vi "2d 10Be.vi"(6 "data in":T6={"Total counts"=0, "cps"=0.0, "live time"=0.0, "pulser"=0.0, "rare counts"=0.0, "other counts"=0.0, "total run time(sec)"=0.0, "adjusted run time(sec)"=0.0, "17O average"=1.0, "17O current"=1.0}, 8 "error in":errorcluster, 9 "1d state control":T7) -> (4 "data out":T6={"Total counts"=0, "cps"=0.0, "live time"=0.0, "pulser"=0.0, "rare counts"=0.0, "other counts"=0.0, "total run time(sec)"=0.0, "adjusted run time(sec)"=0.0, "17O average"=1.0, "17O current"=1.0})   [LabVIEW 2016]
doc: "uses gated region to gather and parse 1d data"
uses:
  controls/1d/1d state event control.ctl
  spectrum/controls/count control.ctl
  controls/display spectrum.ctl
  pixie2d/controls/1d gate selection.ctl
  <vilib>/DAQmx/read.llb/DAQmx Read (Analog 1D DBL 1Chan NSamp).vi
  <vilib>/Analysis/baseanly.llb/Mean (DBL).vi
  <vilib>/DAQmx/miscellaneous.llb/DAQmx Fill In Error Info.vi
  Drivers/Pixie4DLL.dll
  <vilib>/Analysis/NI_AALBase.lvlib
panel:
  out "number of events":dbl
  out "Run time [s]":dbl
  out "run data output":T1
  in  "wait time(milliseconds)":i32=500
  in  "17O scale (nA/V)":dbl=5.0
  out "17O":dbl
  out "error out":errorcluster
  out "17 Average":dbl format="%0.6f"
  out "17O information":dbl[](array[numeric])
  out "sum  17O":dbl format="%0.2f"
  out "splice time":u32 format="%.2e"
  out "17O":dbl(graph)
  in  "1d gate":T3={"channel number"="", "min"=0.0, "max"=32000.0}
  in  "stop":bool
  in  "number of gated regions":i32=3
  in  "spectrum 2":T4 items=["pulser", "gated region 1", "gated region 2", "gated region 3"]
  in  "spectrum":T4 items=["pulser", "gated region 1", "gated region 2", "gated region 3"]
  out "gate 2":dbl[][](graph)
  out "gate 1":dbl[][](graph)
  out "display array out":T5(array[cluster])
  out "Pixie4DLL calls error":errorcluster
  out "run time":sgl
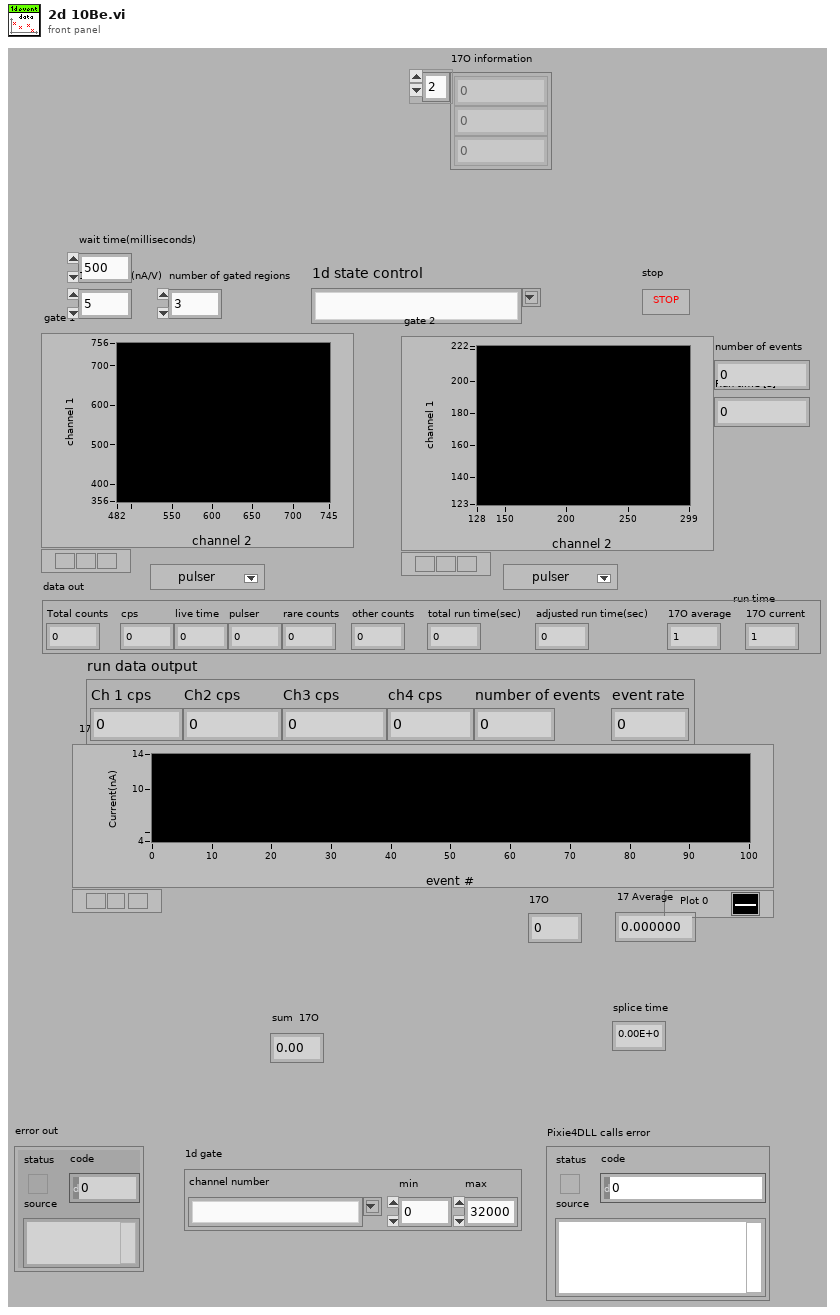
[diagram p1: front panel]
types:
  T1 = cluster{"Ch 1 cps":dbl, "Ch2 cps":dbl, "Ch3 cps":dbl, "ch4 cps":dbl, "number of events":dbl, "event rate":dbl}
  T2 = typedef "1d gate selection.ctl" = string
  T3 = cluster{"channel number":T2, "min":dbl, "max":dbl}
  T4 = typedef "display spectrum.ctl" = u16
  T5 = cluster{"X name":string, "Y name ":string, "counts":dbl, "gate 1":dbl[][], "count rate":dbl, "X Peak":dbl, "Y Peak":dbl, "cathode position":dbl}[]
  T6 = typedef "count control.ctl" = cluster{"Total counts":u32, "cps":dbl, "live time":dbl, "pulser":dbl, "rare counts":dbl, "other counts":dbl, "total run time(sec)":dbl, "adjusted run time(sec)":dbl, "17O average":dbl, "17O current":dbl}
  T7 = typedef "1d state event control.ctl" = string
  T8 = cluster{"X name":string, "Y name ":string, "counts":dbl, "gate 1":dbl[][], "count rate":dbl, "X Peak":dbl, "Y Peak":dbl, "cathode position":dbl}
  T9 = cluster{"input count rate 0":dbl, "input count rate 1":dbl, "input count rate 2":dbl, "input count rate 3":dbl, "number of events":dbl, "event rate":dbl}
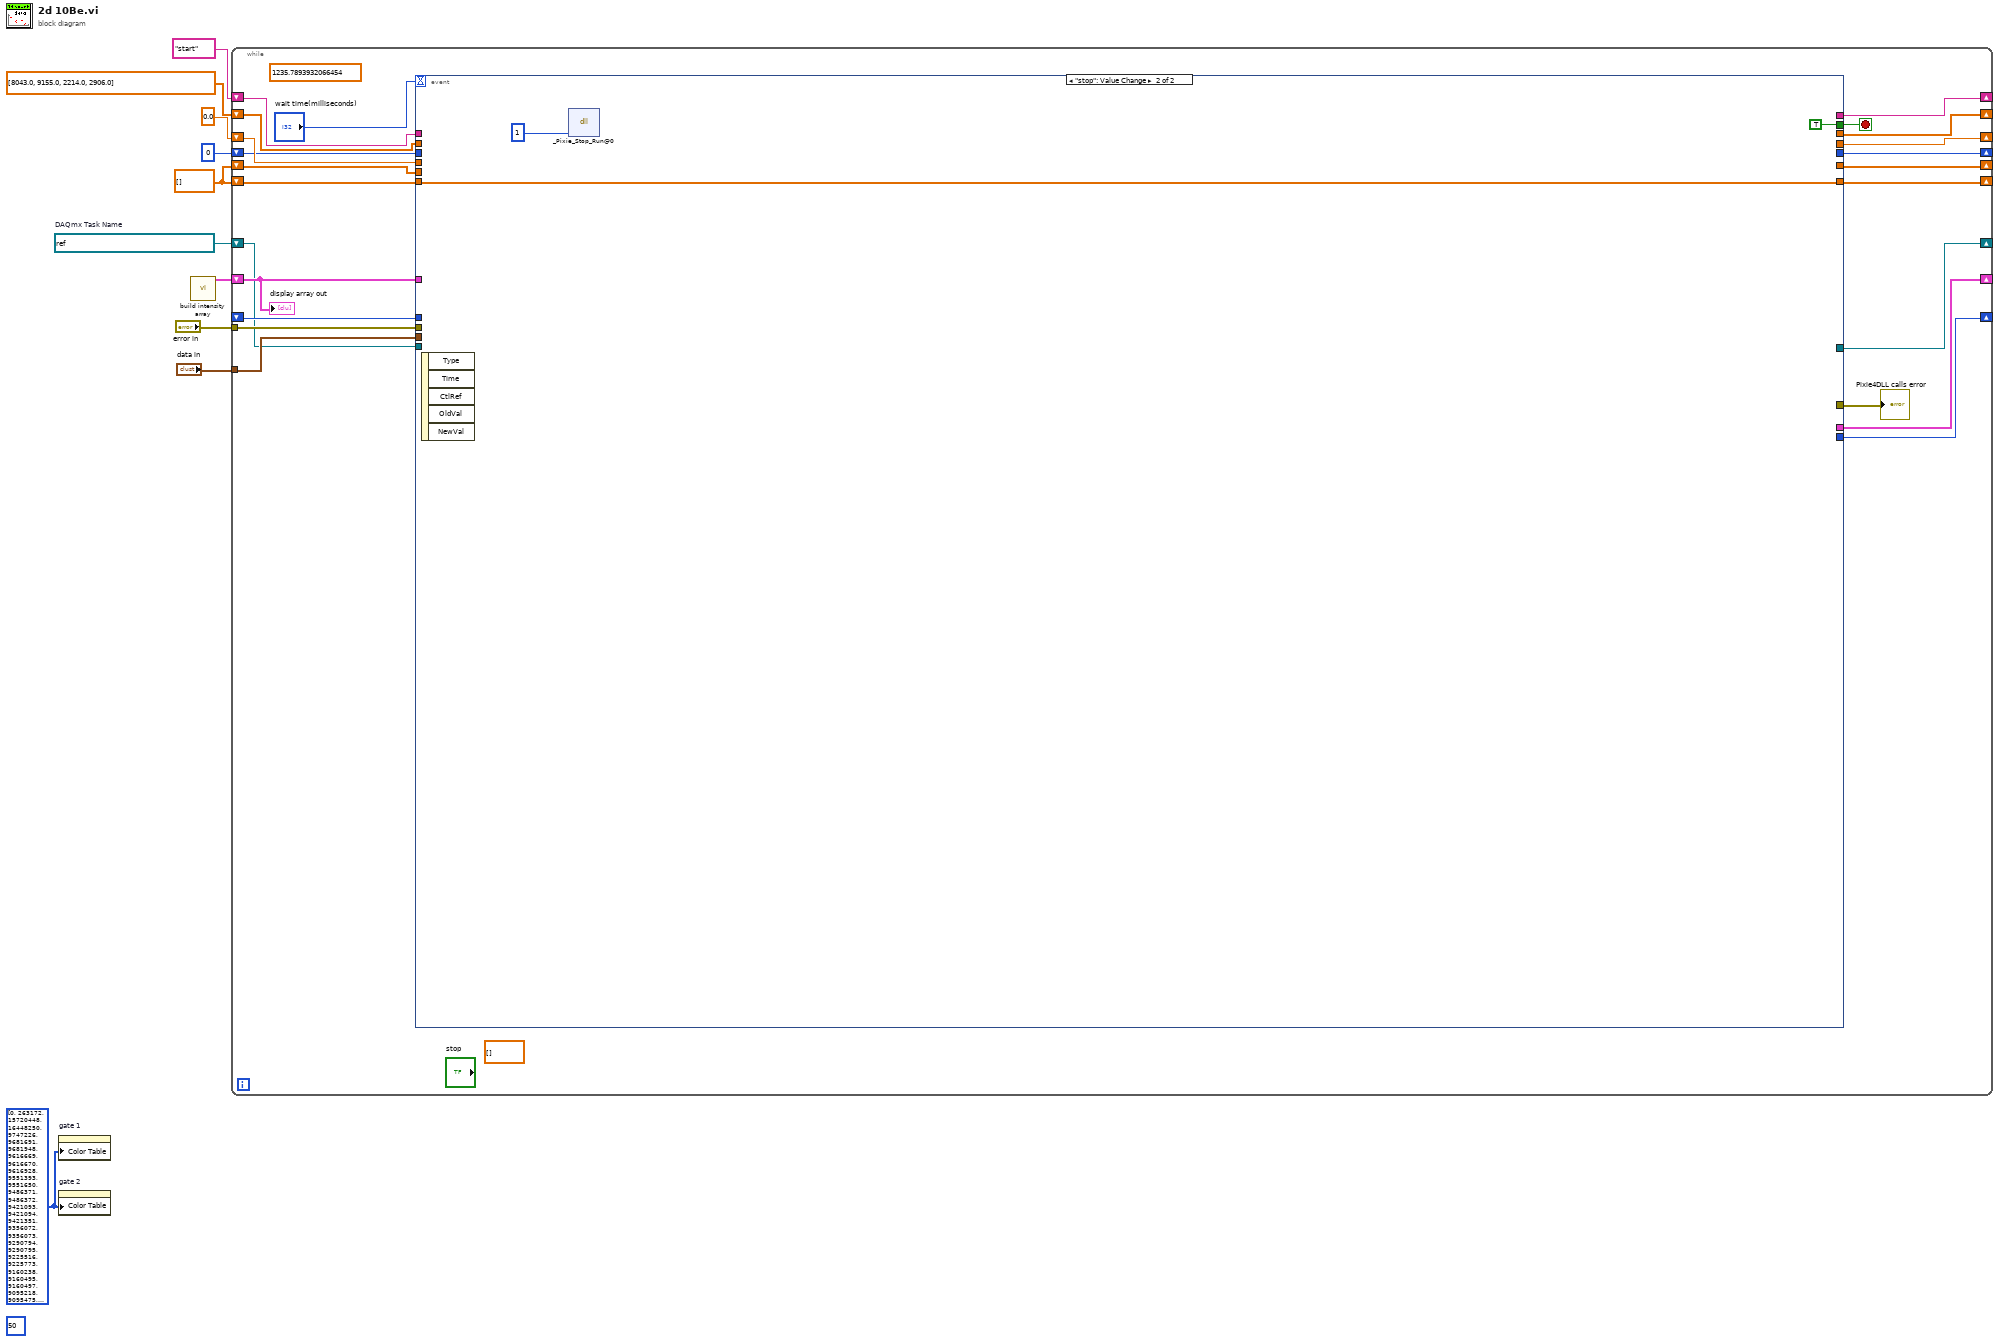
[diagram p0: block diagram]
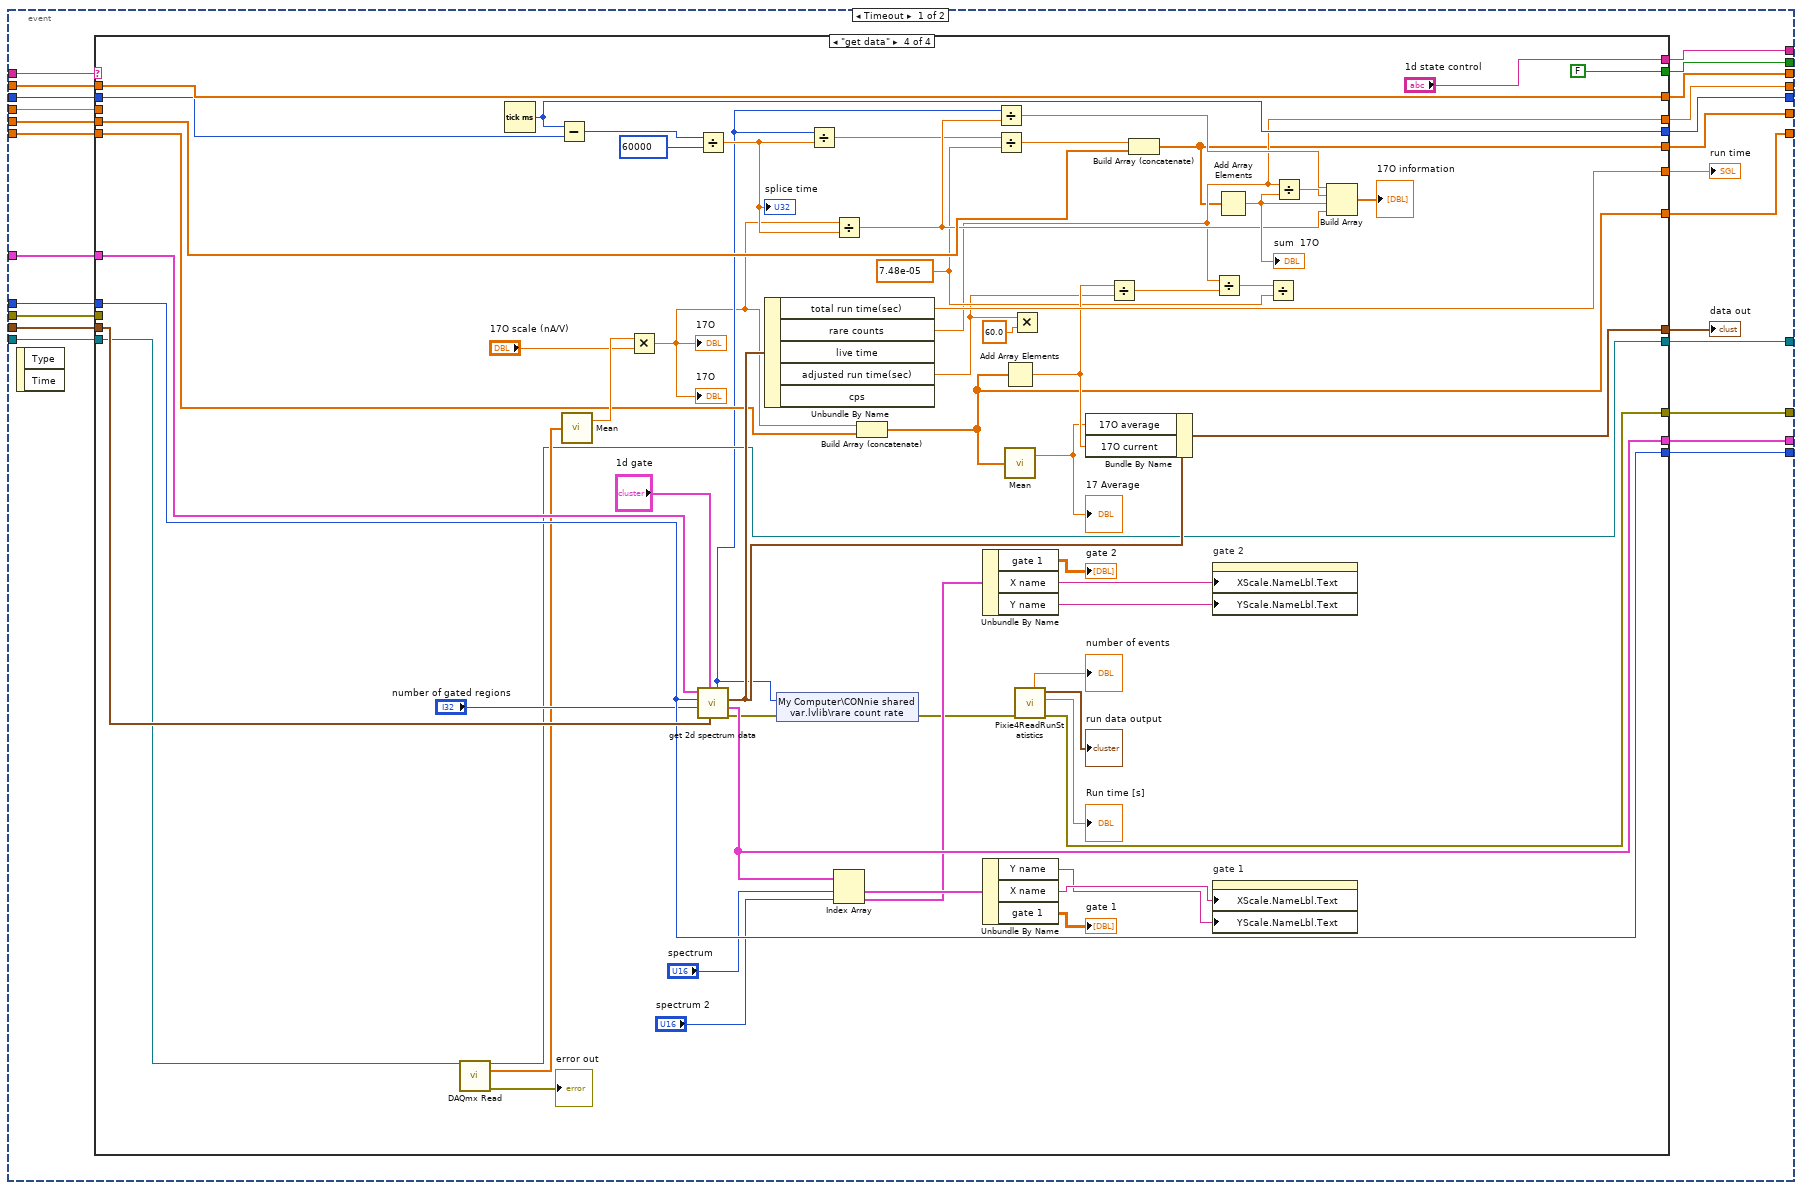
[diagram p2: hidden frame]
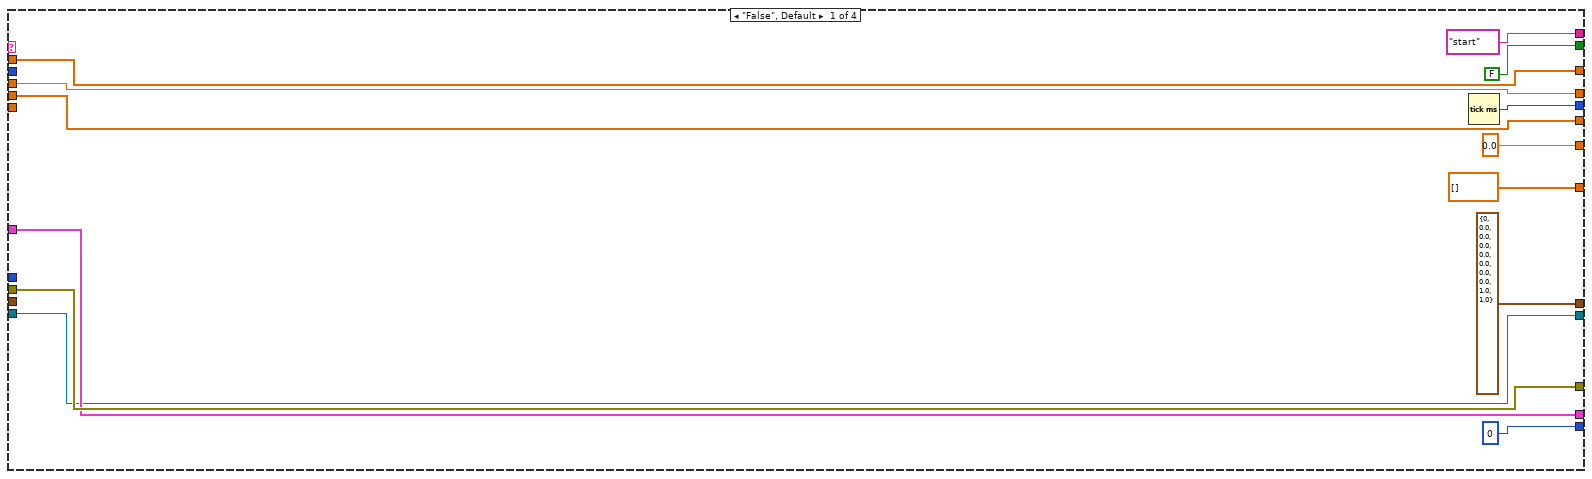
[diagram p3: hidden frame]
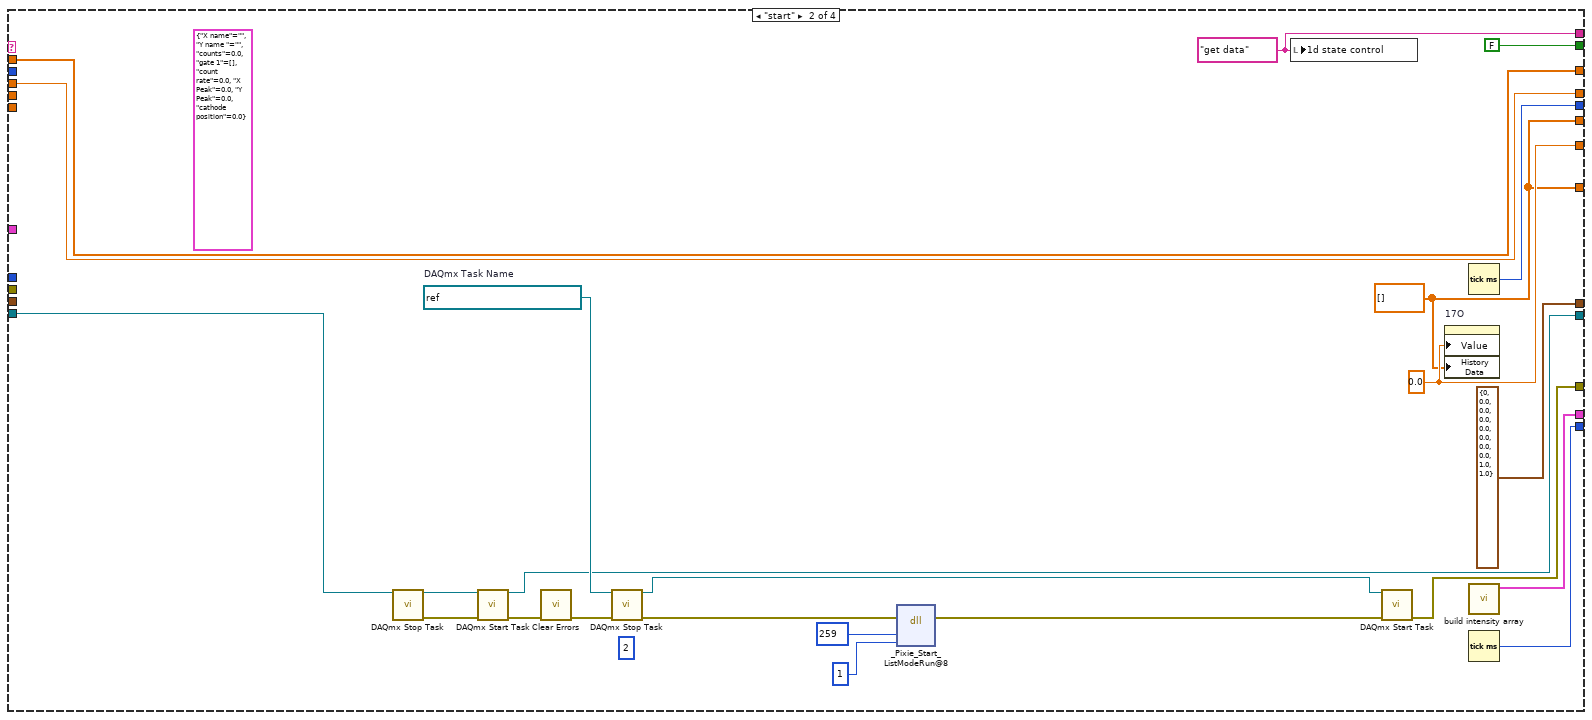
[diagram p4: hidden frame]
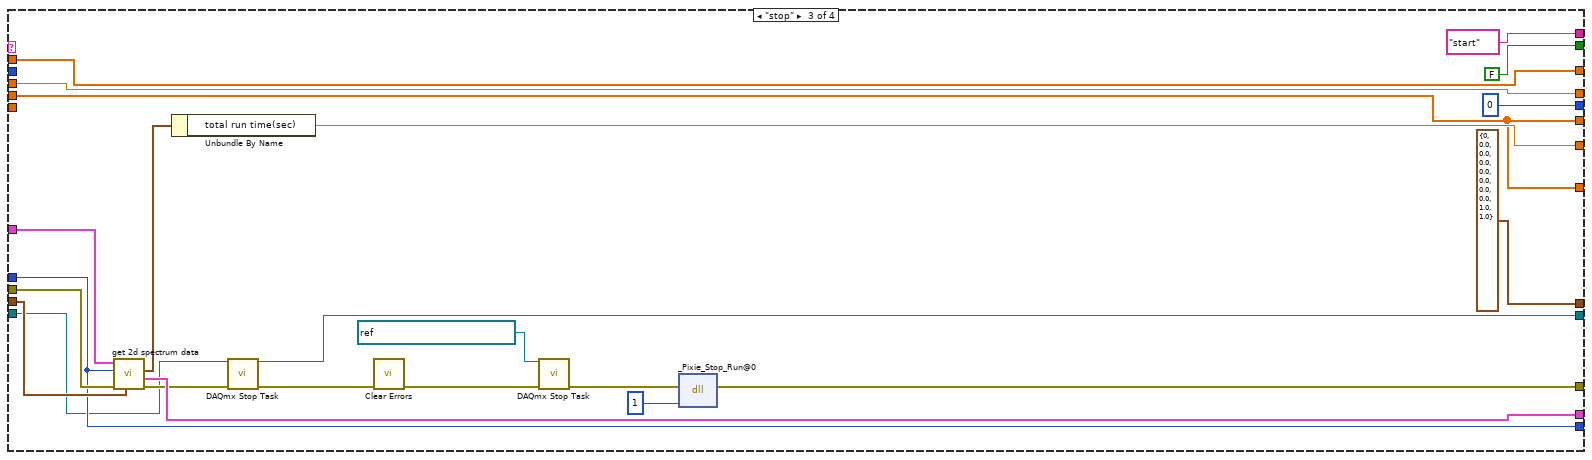
[diagram p5: hidden frame]
diagram:
  w1 = dbl[] []
  w3 = refnum<k21> "measure constant voltage"  # DAQmx Task Name
  w5 = u32[] [0, 263172, 15720448, 16448250, 9747226, 9681691, 9681948, 9616669, 9616670, 9616928, 9551393, 9551650, 9486371, 9486372, 9421093, 9421094, 9421351, 9356072, 9356073, 9290794, 9290795, 9225516, 9225773, 9160238, 9160495, 9160497, 9095218, 9095475, 9029940, 9030197, 8964918, 8964919, 8965176, 8899641, 8899898, 8834619, 8834620, 8769341, 8769342, 8769599, 8704321, 8704322, 8639043, 8639044, 8573765, 8574022, 8574023, 8508744, 8508745, 8443466, 8443723, 8378188, 8378445, 8312910, 8313167, 8312912, 8247122, 8246867, 8181076, 8181077, 8115286, 8115031, 8114776, 8048985, 8048730, 7982939, 7982684, 7916893, 7916894, 7916639, 7850848, 7850594, 7784803, 7784548, 7718757, 7718502, 7718503, 7652712, 7652457, 7586666, 7586411, 7520620, 7520365, 7454574, 7454319, 7454320, 7388529, 7388275, 7322484, 7322229, 7256438, 7256183, 7255928, 7190137, 7190138, 7124347, 7124092, 7058301, 7058046, 7057791, 6992000, 6991745, 6926211, 6925956, 6860165, 6859910, 6859655, 6793864, 6793609, 6727818, 6727563, 6662028, 6661773, 6595982, 6595727, 6595472, 6529681, 6529426, 6463636, 6463381, 6397846, 6397591, 6397336, 6331545, 6331290, 6265499, 6265243, 6199451, 6199451, 6199195, 6133403, 6133147, 6067355, 6067100, 6001308, 6001052, 6000796, 5935260, 5935004, 5869212, 5868956, 5803164, 5802908, 5737116, 5736860, 5736604, 5671068, 5670813, 5605021, 5604765, 5538973, 5538717, 5538461, 5472669, 5472413, 5406877, 5406621, 5340829, 5340573, 5340317, 5274525, 5274270, 5208478, 5208478, 5142686, 5142430, 5142174, 5076382, 5076126, 5010334, 5010078, 4944286, 4944286, 4878494, 4878238, 4877982, 4812191, 4811935, 4746143, 4745887, 4680095, 4680095, 4679839, 4614047, 4613791, 4547999, 4547743, 4481951, 4481695, 4678303, 4874656, 5005472, 5201824, 5398176, 5594528, 5790880, 5987232, 6183584, 6314656, 6511008, 6707360, 6903712, 7100064, 7230880, 7427233, 7623585, 7819937, 8016545, 8212897, 8409249, 8540065, 8736417, 8932769, 9129121, 9325473, 9456545, 9652897, 9849249, 10045601, 10241954, 10438306, 10634658, 10765474, 10961826, 11158434, 11354786, 11551138, 11681954, 11878306, 12074658, 12271010, 12467362, 12663714, 12860323, 12991139, 13187491, 13383843, 13580195, 13776547, 13907363, 14103715, 14300323, 14496675, 14693027, 14889379, 15085731, 15216547, 15412900, 15609252, 15805604, 16002212, 16133028, 16329380, 16525732, 16722084, 16711680, 16448250, 16448250, 16448250]
  (unwired) 50
  n1 = property on="gate 1" class="IntGraph (strict)"("Color Table"=w5) -> ()  [unwired: 2 in, 2 out]
  n2 = property on="gate 2" class="IntGraph (strict)"("Color Table"=w5) -> ()  [unwired: 2 in, 2 out]
  n3 = call "build intensity array.vi"() -> ("display array out"=w6:T5)  [unwired: 10 in, 1 out]
  n4 = while {
    tunnel: "error in" -> [w31]
    tunnel: "data in" -> [w30]
    shift-right: [w29] -> _
    shift-left: _ -> [w33]
    shift-right: [w25] -> _
    shift-left: dbl[] [8043.0, 9155.0, 2214.0, 2906.0] ("Array 2") -> [w32]
    shift-right: [w23] -> _
    shift-left: T7 "start" ("1d state control") -> [w28]
    shift-right: [w22] -> _
    shift-left: w6 -> [w21]
    shift-right: [w20] -> _
    shift-left: 0.0 ("total run time(sec)") -> [w19]
    shift-right: [w17] -> _
    shift-left: w3 -> [w18]
    shift-right: [w11] -> _
    shift-left: u32 0 ("millisecond timer value") -> [w16]
    shift-right: [w15] -> _
    shift-left: w1 -> [w14]
    shift-right: [w13] -> _
    shift-left: w1 -> [w12]
    stop <- w27 stop-if-true
    (unwired) dbl[] []
    (unwired) 1235.7893932066454 ("element")
    n5 = event shown="[1] \"stop\": Value Change" {
      selector: _ -> [_ _]
      dyn-events: _ -> [_ _]
      timeout: "wait time(milliseconds)" -> [_ _]
      tunnel: w33 -> [w57 _]
      tunnel: w32 -> [w55 _]
      tunnel: w31 -> [w54 _]
      tunnel: w30 -> [w53 _]
      tunnel: [w52 _] -> w29
      tunnel: [w51 _] -> w25
      tunnel: w28 -> [w50 _]
      tunnel: [w47 TRUE ("stop")] -> w27
      tunnel: [w49 _] -> w26
      tunnel: [w46 _] -> w23
      tunnel: [w45 _] -> w22
      tunnel: w21 -> [w44 _]
      tunnel: [w43 _] -> w20
      tunnel: w19 -> [w42 _]
      tunnel: w18 -> [w41 _]
      tunnel: [w40 _] -> w17
      tunnel: [w39 _] -> w11
      tunnel: w16 -> [w38 _]
      tunnel: [w37 _] -> w15
      tunnel: w14 -> [w36 _]
      tunnel: [w35 w177] -> w13
      tunnel: w12 -> [w34 w177]
      event Timeout {
        n6 = event-data() -> ()  [unwired: 1 in, 2 out]
        n7 = case shown="\"get data\"" w50 {
          tunnel: w57 -> [_ _ w112 w175]
          tunnel: [0.0 w72 w115 w157] -> w56
          tunnel: w55 -> [w68 w92 w111 w174]
          tunnel: [T6 {"Total counts"=0, "cps"=0.0, "live time"=0.0, "pulser"=0.0, "rare counts"=0.0, "other counts"=0.0, "total run time(sec)"=0.0, "adjusted run time(sec)"=0.0, "17O average"=1.0, "17O current"=1.0} ("data in") T6 {"Total counts"=0, "cps"=0.0, "live time"=0.0, "pulser"=0.0, "rare counts"=0.0, "other counts"=0.0, "total run time(sec)"=0.0, "adjusted run time(sec)"=0.0, "17O average"=1.0, "17O current"=1.0} ("data in") T6 {"Total counts"=0, "cps"=0.0, "live time"=0.0, "pulser"=0.0, "rare counts"=0.0, "other counts"=0.0, "total run time(sec)"=0.0, "adjusted run time(sec)"=0.0, "17O average"=1.0, "17O current"=1.0} ("data in") w145] -> w48
          tunnel: w54 -> [w67 _ w114 _]
          tunnel: w53 -> [_ _ w113 w176]
          tunnel: [u32 0 ("millisecond timer value") w93 w112 w175] -> w52
          tunnel: [w68 w92 w111 w174] -> w51
          tunnel: [w67 w87 w106 w120] -> w49
          tunnel: [FALSE ("stop") FALSE ("stop") FALSE ("stop") FALSE ("stop")] -> w47
          tunnel: [T7 "start" ("1d state control") w89 T7 "start" ("1d state control") "1d state control"] -> w46
          tunnel: [w63 w81 w103 w170] -> w45
          tunnel: w44 -> [w63 _ w102 w171]
          tunnel: [w62 w80 w101 w130] -> w43
          tunnel: w42 -> [w62 w80 w101 _]
          tunnel: w41 -> [w61 w77 w96 w155]
          tunnel: [w61 w76 w97 w142] -> w40
          tunnel: [w60 w73 u32 0 ("millisecond timer value") w144] -> w39
          tunnel: w38 -> [_ _ _ w154]
          tunnel: [w59 w71 w94 w126] -> w37
          tunnel: w36 -> [w59 _ w94 w153]
          tunnel: [dbl[] [] w71 w94 w124] -> w35
          tunnel: w34 -> [_ _ _ w138]
          frame "False", Default {
            n8 = Tick Count (ms)() -> (millisecond timer value=w60:u32)
          }
          frame "start" {
            w71 = dbl[] []
            (unwired) T8 {"X name"="", "Y name "="", "counts"=0.0, "gate 1"=[], "count rate"=0.0, "X Peak"=0.0, "Y Peak"=0.0, "cathode position"=0.0} ("xy position cluster")
            (unwired) 2 ("index")
            w88 = refnum<k21> "MyCountEdgesTask"  # DAQmx Task Name
            w89 = T7 "get data" ("1d state control")
            w72 = 0.0
            n9 = call <vilib>:"DAQmx Stop Task.vi"("task/channels in"=w77) -> ("task out"=w78:refnum<k21>, "error out"=w79:errorcluster)  [unwired: 13 in]
            n10 = call <vilib>:"DAQmx Start Task.vi"("task/channels in"=w78, "error in"=w79) -> ("task out"=w76:refnum<k21>, "error out"=w75:errorcluster)  [unwired: 12 in]
            n11 = call <vilib>:"Clear Errors.vi"("error in (no error)"=w75) -> ("error out"=w74:errorcluster)  [unwired: 5 in, 1 out]
            n12 = call <vilib>:"DAQmx Stop Task.vi"("task/channels in"=w88, "error in"=w74) -> ("task out"=w84:refnum<k21>, "error out"=w83:errorcluster)  [unwired: 12 in]
            n13 = dll-call lib="D:/Repo/PRIME Lab 2017a/DAQuiri/PRIME DAQ 2017a/Drivers/Pixie4DLL.dll" fn="_Pixie_Start_ListModeRun@8"(error in=w83, "Run_Type"=u16 259, "Mode"=1) -> (error out=w82:errorcluster)  [unwired: 2 in, 4 out]
            n14 = local write "1d state control"(w89) -> ()
            n15 = call <vilib>:"DAQmx Start Task.vi"("task/channels in"=w84, "error in"=w82) -> ("error out"=w87:errorcluster)  [unwired: 12 in, 1 out]
            n16 = property on="17O" class="WFChart (strict)"("Value"=w72, "History Data"=w71) -> ()  [unwired: 2 in, 2 out]
            n17 = Tick Count (ms)() -> (millisecond timer value=w73:u32)
            n18 = call "build intensity array.vi"() -> ("display array out"=w81:T5)  [unwired: 10 in, 1 out]
            n19 = Tick Count (ms)() -> (millisecond timer value=w93:u32)
          }
          frame "stop" {
            n20 = call "get 2d spectrum data.vi"("data in"=w113, "error in"=w114, "time in"=w112, "display array in"=w102) -> ("error out"=w100:errorcluster, "display array out"=w103:T5, "data out"=w105:T6)  [unwired: 2 in, 3 out]
            n21 = Unbundle By Name(w105) -> ("total run time(sec)"=w115:dbl)
            n22 = call <vilib>:"DAQmx Stop Task.vi"("task/channels in"=w96, "error in"=w100) -> ("task out"=w97:refnum<k21>, "error out"=w99:errorcluster)  [unwired: 12 in]
            n23 = call <vilib>:"Clear Errors.vi"("error in (no error)"=w99) -> ("error out"=w98:errorcluster)  [unwired: 5 in, 1 out]
            n24 = call <vilib>:"DAQmx Stop Task.vi"("task/channels in"=refnum<k21> "MyCountEdgesTask", "error in"=w98) -> ("error out"=w107:errorcluster)  [unwired: 12 in, 1 out]
            n25 = dll-call lib="D:/Repo/PRIME Lab 2017a/DAQuiri/PRIME DAQ 2017a/Drivers/Pixie4DLL.dll" fn="_Pixie_Stop_Run@0"(error in=w107, "mode"=u16 1 ("ModNum")) -> (error out=w106:errorcluster)  [unwired: 4 in, 1 out]
          }
          frame "get data" {
            w133 = 7.48e-05 ("y")
            n26 = call-poly <vilib>:"DAQmx Read.vi"("task/channels in"=w155) -> ("task out"=w142:refnum<k21>, "data"=w143:dbl[], "error out"=→"error out":errorcluster)  [unwired: 12 in]
            n27 = Tick Count (ms)() -> (millisecond timer value=w144:u32)
            n28 = Subtract(x=w144, y=w154) -> (x-y=w150:u32)
            n29 = call-poly <vilib>:"Mean.vi"("X"=w143) -> ("mean"=w141:dbl)  [unwired: 1 out]
            n30 = Multiply(x=w141, y="17O scale (nA/V)") -> (x*y=w122:dbl)
            "17O" <- w122
            "17O" <- w122
            n31 = Divide(x=w150, y=u32 60000 ("x")) -> (x/y=w137:dbl)
            "splice time" <- w137
            n32 = call "get 2d spectrum data.vi"("data in"=w176, "Cluster"="1d gate", "number of gated regions"="number of gated regions", "time in"=w175, "display array in"=w171) -> ("error out"=w165:errorcluster, "display array out"=w170:T5, "data out"=w148:T6, "counts"=w136:u32)  [unwired: 1 in, 2 out]
            n33 = Unbundle By Name(w148) -> ("total run time(sec)"=w157:dbl, "rare counts"=w130:dbl, "adjusted run time(sec)"=w128:dbl)  [unwired: 2 out]
            n34 = shared-variable "My Computer\\CONnie shared var.lvlib\\rare count rate"(w136, error in=w165) -> (error out=w121:errorcluster)
            n35 = Divide(x=w136, y=w137) -> (x/y=w135:dbl)
            n36 = Divide(x=w122, y=w137) -> (x/y=w139:dbl)
            n37 = Index Array(array=w170, index #1="spectrum", index #2="spectrum 2") -> (element #1=w169:T8, element #2=w168:T8)
            n38 = Build Array (concatenate)(w122, w138) -> (w124:dbl[])
            n39 = Unbundle By Name(w168) -> ("gate 1"=→"gate 2":dbl[][], "X name"=w159:string, "Y name"=w158:string)
            n40 = Unbundle By Name(w169) -> ("Y name"=w160:string, "X name"=w161:string, "gate 1"=→"gate 1":dbl[][])
            n41 = Divide(x=w136, y=w139) -> (x/y=w152:dbl)
            n42 = Divide(x=w135, y=w133) -> (x/y=w127:dbl)
            n43 = Add Array Elements(numeric array=w124) -> (sum=w134:dbl)
            n44 = call-poly <vilib>:"Mean.vi"("X"=w124) -> ("mean"=w123:dbl)  [unwired: 1 out]
            "17 Average" <- w123
            n45 = Multiply(x=w128, y=60.0) -> ()  [unwired: 1 out]
            n46 = call "Pixie4ReadRunStatistics.vi"("error in (no error)"=w121) -> ("error out"=w120:errorcluster, "Run time [s]"=→"Run time [s]":dbl, "run data output"=→"run data output":T9, "number of events"=→"number of events":dbl)  [unwired: 7 in]
            n47 = Bundle By Name(cluster=w148, "17O average"=w123, "17O current"=w134) -> (w145:T6)
            n48 = Divide(x=w134, y=w128) -> (x/y=w132:dbl)
            n49 = Build Array (concatenate)(w127, w153) -> (w126:dbl[])
            n50 = property on="gate 2" class="IntGraph (strict)"("XScale.NameLbl.Text"=w159, "YScale.NameLbl.Text"=w158) -> ()  [unwired: 2 in, 2 out]
            n51 = property on="gate 1" class="IntGraph (strict)"("XScale.NameLbl.Text"=w161, "YScale.NameLbl.Text"=w160) -> ()  [unwired: 2 in, 2 out]
            n52 = Divide(x=w130, y=w132) -> (x/y=w131:dbl)
            n53 = Add Array Elements(numeric array=w126) -> (sum=w147:dbl)
            "sum  17O" <- w147
            n54 = Divide(x=w131, y=w133) -> ()  [unwired: 1 out]
            n55 = Divide(x=w130, y=w147) -> (x/y=w146:dbl)
            n56 = Build Array(w152, w146, w147, w139) -> (→"17O information":dbl[])
          }
        }
        "run time" <- w56
        "data out" <- w48
      }
      event "stop": Value Change {
        n57 = event-data() -> ()  [unwired: 1 in, 5 out]
        n58 = dll-call lib="D:/Repo/PRIME Lab 2017a/DAQuiri/PRIME DAQ 2017a/Drivers/Pixie4DLL.dll" fn="_Pixie_Stop_Run@0"("mode"=u16 1 ("ModNum")) -> ()  [unwired: 5 in, 2 out]
      }
    }
    "Pixie4DLL calls error" <- w26
    "display array out" <- w21
  }
